vi "2_DeepLTK_Boolean_Logic(Inference).vi"() -> ()   [LabVIEW 2020]
uses:
  <vilib>/Ngene/DeepLTK/Toolkit/NN_Network/Controls/NN_Save_Before_Destroy_Options.ctl
  <vilib>/Ngene/DeepLTK/Toolkit/NN_Layers/Layers/Input/API/NN_Layer_Set_Out(Input1D_idx).vi
  <vilib>/Ngene/DeepLTK/Toolkit/Deep_Learning_Toolkit_by_Ngene.lvlib
panel:
  out "Output":bool
  in  "stop":bool
  in  "Input2":bool
  in  "Input1":bool
  in  "Weight File Path":path
  in  "CFG File Path":path
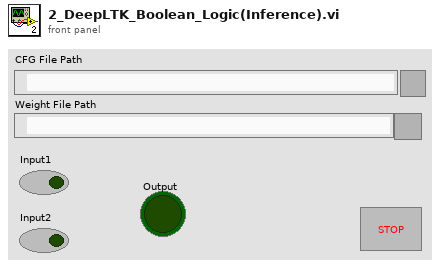
[diagram p1: front panel]
types:
  T1 = typedef "Deep_Learning_Toolkit_by_Ngene.lvlib/NN_Save_Before_Destroy_Options.ctl" = cluster{"CFG?":bool, "Weights?":bool, "Render?":bool}
  T2 = typedef "Deep_Learning_Toolkit_by_Ngene.lvlib/NN_Config_Params.ctl" = cluster{"Name":string, "mBatch":i32, "NN_Train_Params":T3, "LR_Decay_Policy":T6, "Labels":string[], "Loss":T8}
  T3 = typedef "Deep_Learning_Toolkit_by_Ngene.lvlib/NN_Train_Params.ctl" = cluster{"Optimizer":T4, "Beta_1":sgl, "Beta_2":sgl, "Weight Decay(L1)":sgl, "Weight Decay(L2)":sgl, "Data_Sampling":T5}
  T4 = typedef "Deep_Learning_Toolkit_by_Ngene.lvlib/NN_Train_Optimizer.ctl" = enum16{"SGD", "Adam", "Adagrad", "Adadelta", "RMSProp", "Nesterov"}
  T5 = typedef "Deep_Learning_Toolkit_by_Ngene.lvlib/NN_Train_Data_Sampling.ctl" = enum16{"Random", "Sequential"}
  T6 = typedef "Deep_Learning_Toolkit_by_Ngene.lvlib/NN_LR_Policy_Cfg.ctl" = cluster{"Policy_Type":T7, "LR0":dbl, "k":sgl, "WarmUp_Policy":enum16{"Step", "Ramp"}, "WarmUp_Iter":i32, "WarmUp_Ratio":sgl}
  T7 = typedef "Deep_Learning_Toolkit_by_Ngene.lvlib/NN_LR_Policy_Type.ctl" = enum16{"Manual", "Step", "Exp", "1/t"}
  T8 = typedef "Deep_Learning_Toolkit_by_Ngene.lvlib/NN_Loss_Config_Params.ctl" = cluster{"Loss_Type":T9, "Loss_Conf_Params":variant}
  T9 = typedef "Deep_Learning_Toolkit_by_Ngene.lvlib/NN_Loss_Type.ctl" = enum16{"None", "MSE", "CrossEntropy", "YOLO_v2"}
  T10 = typedef "Deep_Learning_Toolkit_by_Ngene.lvlib/NN_Layer_Config_Params.ctl" = cluster{"Layer_Type":T11, "Layer_Conf_Params":variant}
  T11 = typedef "Deep_Learning_Toolkit_by_Ngene.lvlib/NN_Layer_Type.ctl" = enum16{"Input1D", "Input3D", "Conv2D", "Conv2D_Adv", "MaxPool", "AvgPool", "UpSample", "DropOut3D", "ShortCut", "Concat", "SoftMax3D", "FC", "DropOut", "Softmax", "Flatten", "YOLO_v2", "Unsupported"}
  T12 = typedef "Deep_Learning_Toolkit_by_Ngene.lvlib/NN.ctl" = cluster{"Name":string, "No of Layers":i32, "mBatch":i32, "Layers":T13[], "Dimty":T14, "Dims_In":T15, "Dims_Out":T15, "Working_Dir":path, "Train?":bool, "Train_Params":T3, "LR_Update_Policy":T6, "Session Data":T16, "Ground_truth":T17, "NNg_hdls":T19, "NN_Device":T20, "GPU Id":i32, "Labels":string[], "Receptive Field":T21[], "Loss_Type":T9, "Loss_Cfg_Prms":variant}
  T13 = typedef "Deep_Learning_Toolkit_by_Ngene.lvlib/NN_Layer_ref.ctl" = refnum<data-value>
  T14 = typedef "Deep_Learning_Toolkit_by_Ngene.lvlib/NN_In_Out_Dim-ty.ctl" = enum8{"In1D_Out1D", "In3D_Out1D", "In3D_Out3D", "In3D_OutBBox"}
  T15 = typedef "Deep_Learning_Toolkit_by_Ngene.lvlib/NN_Dims(C,H,W).ctl" = cluster{"C":i32, "H":i32, "W":i32}
  T16 = typedef "Deep_Learning_Toolkit_by_Ngene.lvlib/NN_Train_Session_Data.ctl" = cluster{"Epochs":sgl, "Tot_Iter":i32, "LR":sgl, "LR_iter":i32}
  T17 = typedef "Deep_Learning_Toolkit_by_Ngene.lvlib/NN_Ground_truth.ctl" = cluster{"Y":variant, "Y_idx":T18}
  T18 = typedef "Deep_Learning_Toolkit_by_Ngene.lvlib/NN_Data_ref(1D_I32).ctl" = refnum<data-value>
  T19 = typedef "Deep_Learning_Toolkit_by_Ngene.lvlib/nng_cuda_handles.ctl" = cluster{"cudnn":u64, "cublas":u64, "stream":u64, "curand":u64}
  T20 = typedef "Deep_Learning_Toolkit_by_Ngene.lvlib/NN_Device.ctl" = enum16{"CPU", "GPU"}
  T21 = typedef "Deep_Learning_Toolkit_by_Ngene.lvlib/NN_Dims(V,H).ctl" = cluster{"V":i32, "H":i32}
  T22 = typedef "Deep_Learning_Toolkit_by_Ngene.lvlib/NN_Layer.ctl" = cluster{"Name":string, "Layer_Data":variant, "Layer_Type":T11, "Dims_In":T15, "Layers_In":variant, "Dims_Out":T15, "Layers_Out":variant, "Metrics":T23, "GPU_Data":variant, "mBatch":i32, "NN_Device":T20, "NNg_hdls":T19, "Train?":bool, "Dimty":T24, "RecptField":T25}
  T23 = typedef "Deep_Learning_Toolkit_by_Ngene.lvlib/NN_Layer_Metrics.ctl" = cluster{"Data":dbl, "Params":dbl, "Ops":dbl}
  T24 = typedef "Deep_Learning_Toolkit_by_Ngene.lvlib/NN_Layer_Dimty.ctl" = enum16{"1D", "3D"}
  T25 = typedef "Deep_Learning_Toolkit_by_Ngene.lvlib/NN_Layer_RF_State.ctl" = cluster{"Dims":T21, "J":T21}
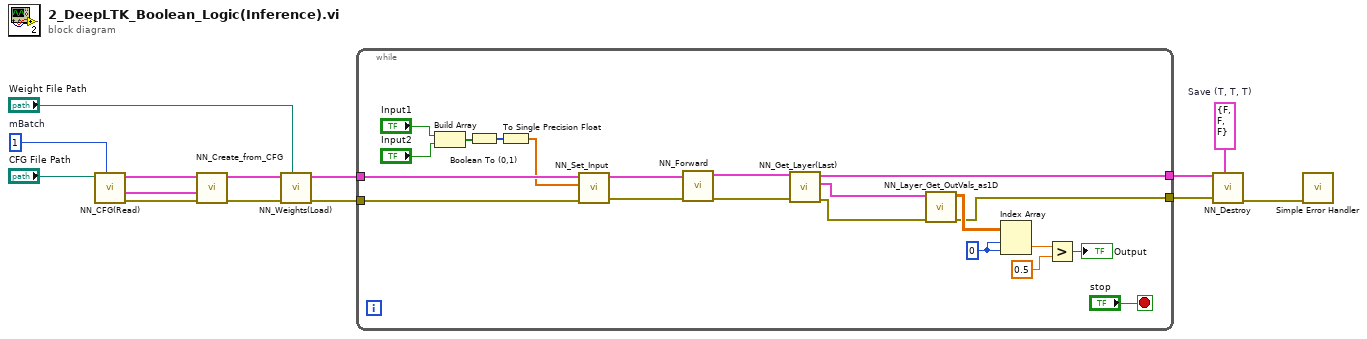
[diagram p0: block diagram]
diagram:
  w2 = T1 {"CFG?"=FALSE, "Weights?"=FALSE, "Render?"=FALSE}  # Save (T, T, T)
  w3 = 1  # mBatch
  n1 = call <vilib>:"NN_CFG(Read).vi"("mBatch"=w3, "CFG file path"="CFG File Path") -> ("error out"=w14:errorcluster, "Net_Cfg"=w4:T2, "Layer_Cfg"=w11:T10[])  [unwired: 7 in]
  n2 = call <vilib>:"NN_Create_from_CFG.vi"("error in (no error)"=w14, "Net_Cfg"=w4, "Layer_Cfg"=w11) -> ("error out"=w13:errorcluster, "NN out"=w12:T12)  [unwired: 7 in]
  n3 = call <vilib>:"NN_Weights(Load).vi"("Weight File Path"="Weight File Path", "error in (no error)"=w13, "NN in"=w12) -> ("error out"=w7:errorcluster, "NN out"=w8:T12)  [unwired: 7 in]
  n4 = while {
    tunnel: w8 -> [w34]
    tunnel: w7 -> [w35]
    tunnel: [w29] -> w6
    tunnel: [w25] -> w5
    stop <- "stop" stop-if-true
    w27 = 0 ("disabled index (col)")
    n5 = Build Array("Input1", "Input2") -> (w26:bool[])
    n6 = Boolean To (0,1)(Boolean=w26) -> (0, 1=w24:i16[])
    n7 = To Single Precision Float(number=w24) -> (single precision float=w23:sgl[])
    n8 = call-poly <vilib>:"NN_Set_Input.vi"("error in (no error)"=w35, "Data_In(1D_SGL)"=w23, "NN In"=w34) -> ("error out"=w32:errorcluster, "NN Out"=w33:T12)  [unwired: 7 in]
    n9 = call <vilib>:"NN_Forward.vi"("error in (no error)"=w32, "NN in"=w33) -> ("error out"=w31:errorcluster, "NN out"=w15:T12)  [unwired: 6 in, 2 out]
    n10 = call <vilib>:"NN_Get_Layer(Last).vi"("error in (no error)"=w31, "NN in"=w15) -> ("error out"=w30:errorcluster, "Last_Layer"=w16:T22, "NN out"=w29:T12)  [unwired: 6 in, 1 out]
    n11 = call <vilib>:"NN_Layer_Get_OutVals_as1D.vi"("error in (no error)"=w30, "Layer"=w16) -> ("error out"=w25:errorcluster, "Out(as1D)"=w28:sgl[][])  [unwired: 8 in]
    n12 = Index Array(array=w28, index (row)=w27, index (col)=w27) -> (element=w19:sgl)
    n13 = Greater?(x=w19, y=sgl 0.5) -> (0:→"Output":bool)
  }
  n14 = call <vilib>:"NN_Destroy.vi"("Save (T, T, T)"=w2, "error in (no error)"=w5, "NN in"=w6) -> ("error out"=w1:errorcluster)  [unwired: 8 in]
  n15 = call <vilib>:"Simple Error Handler.vi"("error in (no error)"=w1) -> ()  [unwired: 4 in, 5 out]
